vi "Specify Delete Action.vi"(11 "Topic in":refnum<class "Topic.lvclass">) -> (2 "Delete action":string, 3 "Topic out":refnum<class "Topic.lvclass">)   [LabVIEW 2015, in "NI_AWS_SNS.lvlib" / "Topic.lvclass"]
uses:
  Topic.lvclass
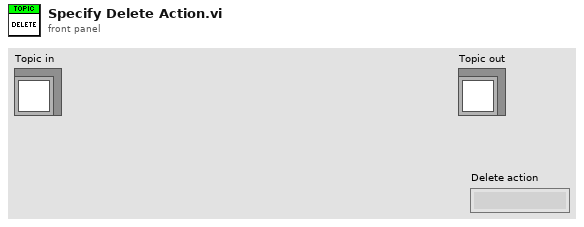
[diagram p1: front panel]
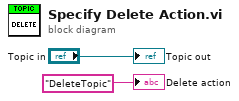
[diagram p0: block diagram]
diagram:
  "Topic out" <- "Topic in"
  "Delete action" <- "DeleteTopic" ("value")
